vi "Tree Map to Tree Control Items.vi"(8 "error in (no error)":errorcluster, 10 "Export Options":T1, 11 "Tree Map Handle In":T5) -> (0 "error out":errorcluster, 3 "Tree Control Items":T10(array[cluster]))   [LabVIEW 2020, in "Blue Tree Map OpenSource.lvlib"]
doc: "Translates the Tree Map representation into Tree Control Elements.\n\n\"Attrible Column Names\" is used to specify the child column data in the tree control. If an attribute isn't found for a tree node, then the data will be blank."
uses:
  Blue Tree Map OpenSource.lvlib
  Typedefs/Tree Map Handle.ctl
  Typedefs/Tree Map.ctl
  Typedefs/Tree Map Data.ctl
  Typedefs/Tree Node Data.ctl
  Typedefs/Attribute Map.ctl
  Typedefs/Tree Map Export Options.ctl
  Typedefs/Tree Map Export Sorting.ctl
  Typedefs/Sort Type.ctl
  Typedefs/Sort AscDesc.ctl
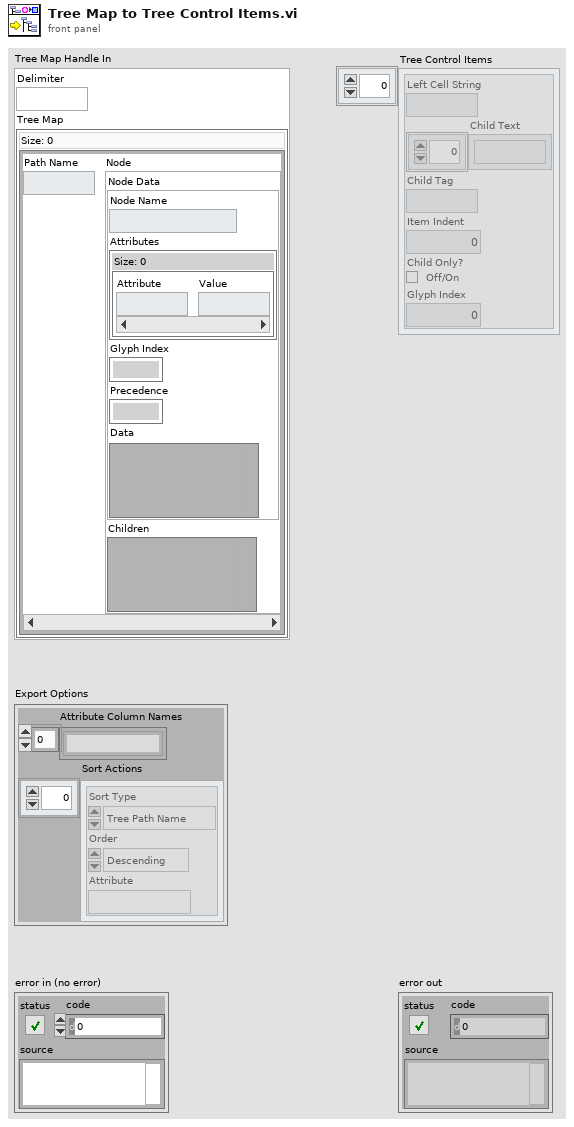
[diagram p1: front panel]
types:
  T1 = typedef "Blue Tree Map OpenSource.lvlib/Tree Map Export Options.ctl" = cluster{"Attribute Column Names":string[], "Sort Actions":T2[]}
  T2 = typedef "Blue Tree Map OpenSource.lvlib/Tree Map Export Sorting.ctl" = cluster{"Sort Type":T3, "Order":T4, "Attribute":string}
  T3 = typedef "Blue Tree Map OpenSource.lvlib/Sort Type.ctl" = enum16{"Tree Path Name", "Node Name", "Attribute", "Precedence"}
  T4 = typedef "Blue Tree Map OpenSource.lvlib/Sort AscDesc.ctl" = enum16{"Descending", "Ascending"}
  T5 = typedef "Blue Tree Map OpenSource.lvlib/Tree Map Handle.ctl" = cluster{"Delimiter":string, "Tree Map":T6}
  T6 = typedef "Blue Tree Map OpenSource.lvlib/Tree Map.ctl" = map{string, T7}
  T7 = typedef "Blue Tree Map OpenSource.lvlib/Tree Map Data.ctl" = cluster{"Node Data":T8, "Children":variant}
  T8 = typedef "Blue Tree Map OpenSource.lvlib/Tree Node Data.ctl" = cluster{"Node Name":string, "Attributes":T9, "Glyph Index":i32, "Precedence":i32, "Data":variant}
  T9 = typedef "Blue Tree Map OpenSource.lvlib/Attribute Map.ctl" = map{string, string}
  T10 = cluster{"Left Cell String":string, "Child Text":string[], "Child Tag":string, "Item Indent":i32, "Child Only?":bool, "Glyph Index":i32}[]
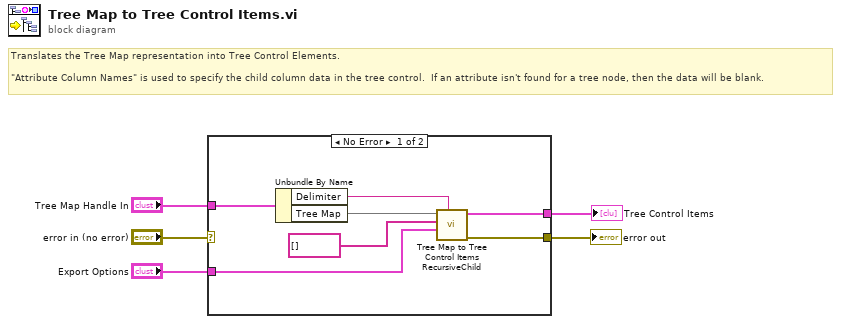
[diagram p0: block diagram]
diagram:
  # "Translates the Tree Map representation into Tree Control Elements.\n\n\"Attribute Column Names\" is used to specify the child column data in the tree control.  If an attribute isn't found for a tree node, then the data will be blank."
  n1 = case shown="No Error" "error in (no error)" {
    selector: "error in (no error)" -> [_ w13]
    tunnel: [w12 _] -> w5
    tunnel: "Export Options" -> [w11 _]
    tunnel: "Tree Map Handle In" -> [w9 _]
    tunnel: [w6 w13] -> w3
    frame No Error {
      n2 = Unbundle By Name(w9) -> ("Delimiter"=w7:string, "Tree Map"=w8:T6)
      n3 = call "Tree Map to Tree Control Items RecursiveChild.vi"("Delimiter"=w7, "Export Options"=w11, "Tree Path (Parent, Child)"=string[] [], "Tree Map In"=w8) -> ("error out"=w6:errorcluster, "Tree Control Item"=w12:T10)  [unwired: 6 in]
    }
    frame Error {
    }
  }
  "Tree Control Items" <- w5
  "error out" <- w3
